vi "Combine Positions by type.vi"(11 "Array in":T2(array[cluster])) -> (3 "Array out":T2(array[cluster]))   [LabVIEW 2019, in "JSONtext.lvlib"]
uses:
  JSONtext.lvlib
  JSON Value Type.ctl
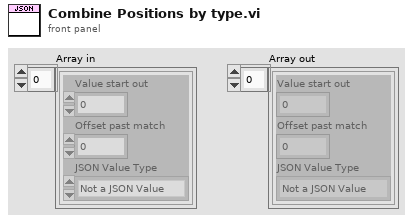
[diagram p1: front panel]
types:
  T1 = typedef "JSONtext.lvlib/JSON Value Type.ctl" = enum16{"Not a JSON Value", "JSON Object", "JSON Array", "String", "Number", "true", "false", "null"}
  T2 = cluster{"Value start out":i32, "Offset past match":i32, "JSON Value Type":T1}[]
  T3 = cluster{"Value start out":i32, "Offset past match":i32, "JSON Value Type":T1}
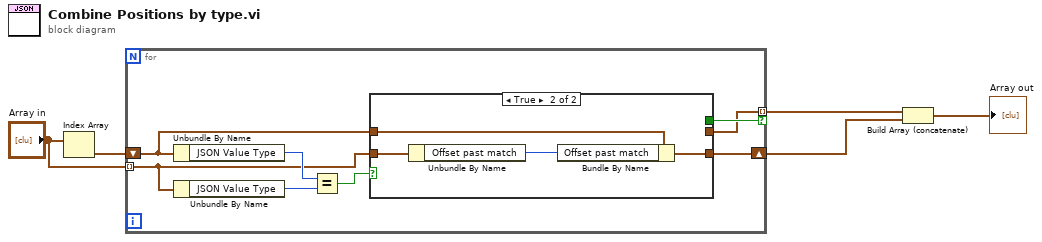
[diagram p0: block diagram]
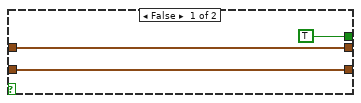
[diagram p2: hidden frame]
diagram:
  n1 = Index Array(array="Array in") -> (element=w2:T3)  [unwired: 1 in]
  n2 = for {
    tunnel: "Array in" -> [w6] mode=indexing
    shift-right: [w7] -> w4
    shift-left: w2 -> [w9]
    tunnel: [w8] -> w3 mode=indexing if=w10
    n3 = Unbundle By Name(w9) -> ("JSON Value Type"=w12:T1)
    n4 = Unbundle By Name(w6) -> ("JSON Value Type"=w13:T1)
    n5 = Equal?(x=w12, y=w13) -> (x = y?=w11:bool)
    n6 = case shown="True" w11 {
      tunnel: [TRUE _] -> w10
      tunnel: w9 -> [w15 w20]
      tunnel: [w15 _] -> w8
      tunnel: w6 -> [w14 w18]
      tunnel: [w14 w19] -> w7
      frame False {
      }
      frame True {
        n7 = Unbundle By Name(w18) -> ("Offset past match"=w17:i32)
        n8 = Bundle By Name(cluster=w20, "Offset past match"=w17) -> (w19:T3)
      }
    }
  }
  n9 = Build Array (concatenate)(w3, w4) -> (→"Array out":T2)
